vi "Actor Core.vi"(8 "error in":errorcluster, 11 "App in":refnum<class "App.lvclass">) -> (0 "error out":errorcluster, 3 "Actor out":refnum<class "Actor.lvclass">)   [LabVIEW 2016, in "App.lvlib" / "App.lvclass"]
doc: "(<B>Filename</B>: Actor Framework.lvlib:Actor.lvclass:Actor Core.vi)\n\nReceives messages to the actor, reacts to them, and initiates any error handling that may shut the actor down.\n\nDescendant classes may override this VI to append parallel tasks for the actor to complete while it handles messages. Overrides use the Call Parent Method node."
uses:
  App.lvclass
  C:/Program Files/National Instruments/LabVIEW 2016/vi.lib/ActorFramework/Actor/Actor.lvclass
  <vilib>/ActorFramework/Actor/Actor.lvclass
  App.lvclass/App.ctl
  <vilib>/ActorFramework/Actor/Actor.lvclass/Actor.ctl
  <vilib>/ActorFramework/Message Enqueuer/Message Enqueuer.lvclass/Message Enqueuer.ctl
  Dynamic Instrument/Dynamic Instrument/Dynamic Instrument.lvclass/Dynamic Instrument.ctl
  Dynamic Instrument/Dynamic Instrument/Read Instrument Name.vi
  <vilib>/ActorFramework/Message Enqueuer/Init from Existing Queue.vi
  <vilib>/ActorFramework/Message Enqueuer/Enqueue.vi
  <vilib>/ActorFramework/Stop Msg/Stop Msg.lvclass
  C:/Program Files/National Instruments/LabVIEW 2016/vi.lib/ActorFramework/Message/Message.lvclass
  <vilib>/ActorFramework/Message Priority Queue/Priority Enqueue.vi
  <vilib>/ActorFramework/Message Enqueuer/Message Enqueuer.lvclass
  Dynamic Instrument/Dynamic Instrument/Dynamic Instrument.lvclass
panel:
  out "Instruments":string[](array[string])
  out "DAQmx loaded":bool
  in  "Stop Button":bool
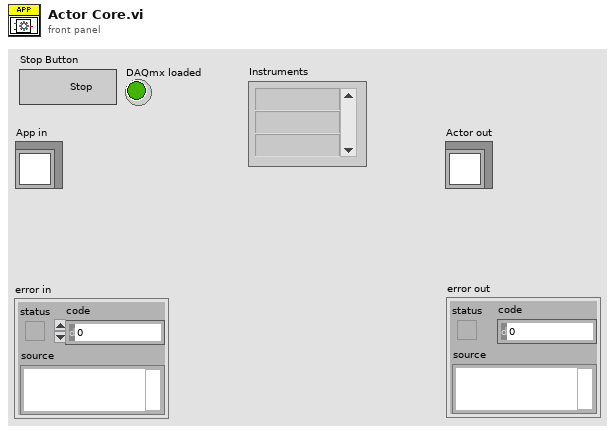
[diagram p1: front panel]
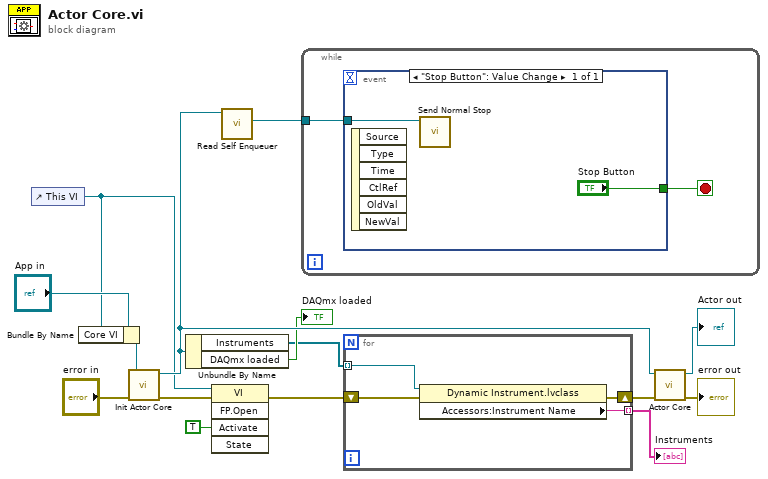
[diagram p0: block diagram]
diagram:
  n1 = control-ref of="This VI"() -> (w1:refnum<vi>)
  n2 = Bundle By Name(cluster="App in", "Core VI"=w1) -> (w2:refnum<class "App.lvclass">)
  n3 = call-dynamic "Init Actor Core.vi"("error in (no error)"="error in", "App in"=w2) -> ("error out"=w4:errorcluster, "App out"=w10:refnum<class "App.lvclass">)  [unwired: 8 in]
  n4 = Unbundle By Name(w10) -> ("Instruments"=w8:refnum<class "Dynamic Instrument.lvclass">[], "DAQmx loaded"=→"DAQmx loaded":bool)
  n5 = invoke class="VI" method="FP.Open"(reference=w1, error in=w4, "Activate"=TRUE ("Activate?")) -> (error out=w3:errorcluster)  [unwired: 2 in, 4 out]
  n6 = call <vilib>:"Read Self Enqueuer.vi"("Actor"=w10) -> ("Self Enqueuer"=w13:refnum<class "Message Enqueuer.lvclass">)  [unwired: 10 in]
  n7 = while {
    tunnel: w13 -> [w16]
    stop <- w17 stop-if-true
    n8 = event shown="[0] \"Stop Button\": Value Change" {
      selector: _ -> [_]
      dyn-events: _ -> [_]
      timeout: _ -> [_]
      tunnel: ["Stop Button"] -> w17
      tunnel: w16 -> [w18]
      event "Stop Button": Value Change {
        n9 = event-data() -> ()  [unwired: 1 in, 6 out]
        n10 = call <vilib>:"Send Normal Stop.vi"("Message Enqueuer"=w18) -> ()  [unwired: 10 in, 1 out]
      }
    }
  }
  n11 = for {
    tunnel: w8 -> [w23] mode=indexing
    tunnel: [w22] -> w7 mode=indexing
    shift-right: [w20] -> w6
    shift-left: w3 -> [w21]
    n12 = property class="Dynamic Instrument.lvclass"(reference=w23, error in=w21) -> (error out=w20:errorcluster, "Accessors:Instrument Name"=w22:string)  [unwired: 1 out]
  }
  "Instruments" <- w7
  n13 = call-parent "Actor Core.vi"("error in"=w6, "Actor in"=w10) -> ("error out"=→"error out":errorcluster, "Actor out"=→"Actor out":refnum<class "Actor.lvclass">)  [unwired: 8 in]
